vi "Wmeter Close.vi"(8 "error in":errorcluster, 11 "WMeter":refnum<visa-resource-name>) -> (0 "error out":errorcluster)   [LabVIEW 2012]
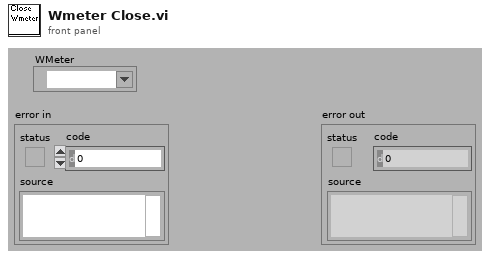
[diagram p1: front panel]
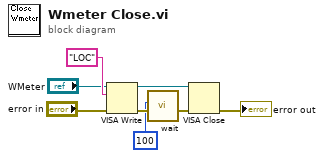
[diagram p0: block diagram]
diagram:
  n1 = VISA Write(VISA resource name="WMeter", write buffer="LOC" ("data"), error in (no error)="error in") -> (VISA resource name out=w1:refnum<visa-resource-name>, error out=w5:errorcluster)  [unwired: 1 out]
  n2 = call "wait.vi"("error in (no error)"=w5, "ms to wait"=u32 100) -> ("error out (no error)"=w4:errorcluster)  [unwired: 7 in]
  n3 = VISA Close(VISA resource name=w1, error in (no error)=w4) -> (error out=→"error out":errorcluster)
